vi "ByteArray2Integer.vi"(1 "Byte Array":u8[](array[numeric])) -> (0 "Integer":u32)   [LabVIEW 2016, in "Brooks MFC.lvclass"]
uses:
  Brooks MFC.lvclass
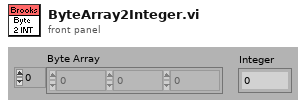
[diagram p1: front panel]
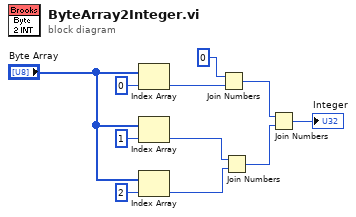
[diagram p0: block diagram]
diagram:
  n1 = Index Array(array="Byte Array", index=0) -> (element=w5:u8)
  n2 = Index Array(array="Byte Array", index=1) -> (element=w6:u8)
  n3 = Index Array(array="Byte Array", index=2) -> (element=w7:u8)
  n4 = Join Numbers(hi=u8 0, lo=w5) -> ((hi.lo)=w3:u16)
  n5 = Join Numbers(hi=w6, lo=w7) -> ((hi.lo)=w2:u16)
  n6 = Join Numbers(hi=w3, lo=w2) -> ((hi.lo)=→"Integer":u32)
